vi "OAT Check Range.vi"(11 "range in":cluster{"start":dbl, "end":dbl, "step":dbl} {"step" format="%.2f"; "end" format="%.2f"; "start" format="%.2f"}) -> (1 "empty?":bool, 2 "num of steps":i32, 3 "range out":cluster{"start":dbl, "end":dbl, "step":dbl} {"step" format="%.2f"; "end" format="%.2f"; "start" format="%.2f"})   [LabVIEW 2017]
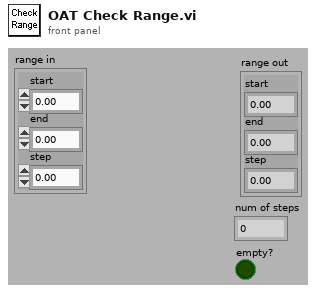
[diagram p1: front panel]
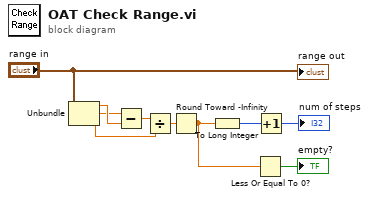
[diagram p0: block diagram]
diagram:
  n1 = Unbundle("range in") -> ("start"=w10:dbl, "end"=w6:dbl, "step"=w8:dbl)
  n2 = Subtract(x=w6, y=w10) -> (x-y=w7:dbl)
  n3 = Divide(x=w7, y=w8) -> (x/y=w9:dbl)
  n4 = Round Toward -Infinity(1:w9) -> (0:w1:dbl)
  n5 = To Long Integer(number=w1) -> (32bit integer=w4:i32)
  n6 = Less Or Equal To 0?(x=w1) -> (x <= 0?=→"empty?":bool)
  n7 = Increment(x=w4) -> (x+1=→"num of steps":i32)
  "range out" <- "range in"
